vi "Callback VI Reference.vi"   [LabVIEW 2021, in "Utilities.lvlib"]
doc: "Maintains a static reference to a callback VI. After you place the Callback VI Reference function on the block diagram, double-click the Callback VI Reference function to display a file dialog box where you can select a callback VI."
uses:
  <vilib>/myRIO/Instrument Drivers/Utilities/Utilities.lvlib
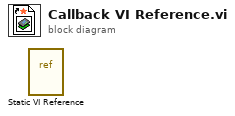
[diagram p0: block diagram]
diagram:
  n1 = vi-ref "Static VI Reference"() -> ()  [unwired: 1 out]
